vi "Send commands to manipulator.vi"(6 "read":bool, 7 "delay before read (ms)":u32, 9 "Commands (microns)":T5 {"Zcommand (nm)" min=0.0 max=25000000.0 step=62.5 format="%.1f"; "Ycommand (nm)" format="%.1f"; "Xcommand (nm)" format="%.1f"}, 10 "Manipulator":i32(ring) items=["1", "2", "3", "4"], 11 "Command":u16(ring)=1 items=["Change manipulator", "Get current position", "Go to position", "Home", "Work", "Center", "Interrupt move"]) -> (0 "Coordinates (not rounded)":T1 {"Zcoordinate (not rounded)" format="%.4f"; "Ycoordinate (not rounded)" format="%.4f"; "Xcoordinate (not rounded)" format="%.4f"}, 1 "Coordinates (microns)":T2={"Xcoordinate (microns)"=8589, "Ycoordinate (microns)"=6028, "Zcoordinate (microns)"=4319}, 2 "Coordinates (nm)":T3={"Xcoordinate (nm)"=8589.0, "Ycoordinate (nm)"=6028.0, "Zcoordinate (nm)"=4319.0} {"Xcoordinate (nm)" format="%.1f"; "Ycoordinate (nm)" format="%.1f"; "Zcoordinate (nm)" format="%.1f"}, 3 "Commands (microns)":T4 {"Zcommand (microns)" format="%.4f"; "Ycommand (microns)" format="%.4f"; "Xcommand (microns)" format="%.4f"}, 5 "Error":bool)   [LabVIEW 2010]
doc: "The Basic Serial Read and Write example performs a Serial Port Read, a Serial Port Write, or a combination of these actions. The user selects the actions (read or write) on the front panel. If both are selected, the VI will write the data first, read data, and then close the VISA session that is opened to the port. This VI will wait until the specified number of bytes is received at the port. Only the number of bytes specified will be read.\n\nINSTRUCTIONS:\n1) Select the serial resource and configuration parameters (baud rate, data bits, parity, stop bits, flow control).\n2) Select the operations to be performed. \n3) Connect the serial port to your device. If no device is available, perform a loopback test by doing one of the following. Short pins 2 and 3 on a RS-232 cable or short pin 4 to pin 8 and pin 5 to pin 9 on a RS-485/422 cable. \n4) Run the VI to see the data read. (The \"read string\" will match the \"string to write\" if a loopback test was performed.)\n\nNote: The parameters set for the serial port must match the parameters of the connected instrument or device. In this example, the bytes to read parameter specifies the number of bytes that the serial port reads. If there were more bytes at the port than the number specified in bytes to read, those bytes would not be read. Also, if you specify to read more bytes than the number of bytes actually read, you might receive a timeout error message.\n\nOn the block diagram, the Configure Serial Port VI sets the configuration parameters. The front panel displays the controls used to configure the basic parameters, such as baud rate, data bits, and parity. Constants configure the other parameters the user probably does not need set. After the VISA Configure Serial Port VI opens the VISA session and configures the port, the VI passes the VISA resource name to other VIs that perform operations on that VISA resource. The VISA Write function sends a command to the serial device and the VISA Read function returns data based on the command. The VISA Close function then closes the reference to the serial device. It is important to close the reference; otherwise communication through with that port through protocols other than VISA might not be possible."
uses:
  <vilib>/Instr/_visa.llb/VISA Configure Serial Port (Instr).vi
panel:
  in  "flow control":u16(ring) items=["None"=0, "XON/XOFF"=1, "RTS/CTS"=2, "DTR/DSR"=4]
  in  "stop bits":u16(ring)=10 items=["1.0"=10, "1.5"=15, "2.0"=20]
  out "string to write":string="C"
  out "bytes read":u32=13
  out "read string":string
  in  "parity":u16(ring) items=["None", "Odd", "Even", "Mark", "Space"]
  in  "data bits":u16=8 min=5 max=8 step=1
  in  "baud rate":u32=128000
  in  "VISA resource name":refnum<visa-resource-name>="COM3"
  # "hex display"
  # "NOTES\n-Smallest step = 1 microstep = .0625 microns = 62.5 nm\n-16 microsteps/micron\n\n-"
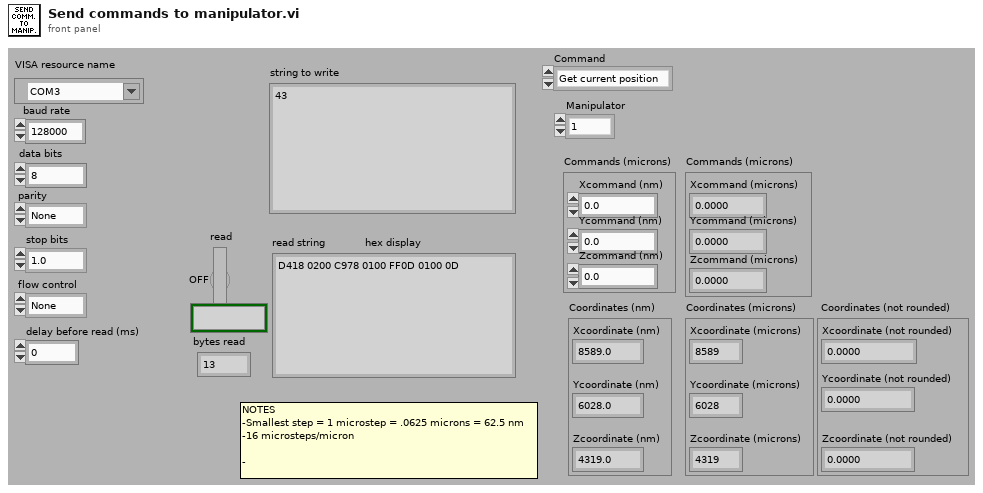
[diagram p1: front panel]
types:
  T1 = cluster{"Xcoordinate (not rounded)":dbl, "Ycoordinate (not rounded)":dbl, "Zcoordinate (not rounded)":dbl}
  T2 = cluster{"Xcoordinate (microns)":i32, "Ycoordinate (microns)":i32, "Zcoordinate (microns)":i32}
  T3 = cluster{"Xcoordinate (nm)":dbl, "Ycoordinate (nm)":dbl, "Zcoordinate (nm)":dbl}
  T4 = cluster{"Xcommand (microns)":dbl, "Ycommand (microns)":dbl, "Zcommand (microns)":dbl}
  T5 = cluster{"Xcommand (nm)":dbl, "Ycommand (nm)":dbl, "Zcommand (nm)":dbl}
  T6 = cluster{"Xcoordinate":i32, "Ycoordinate":i32, "Zcoordinate":i32}
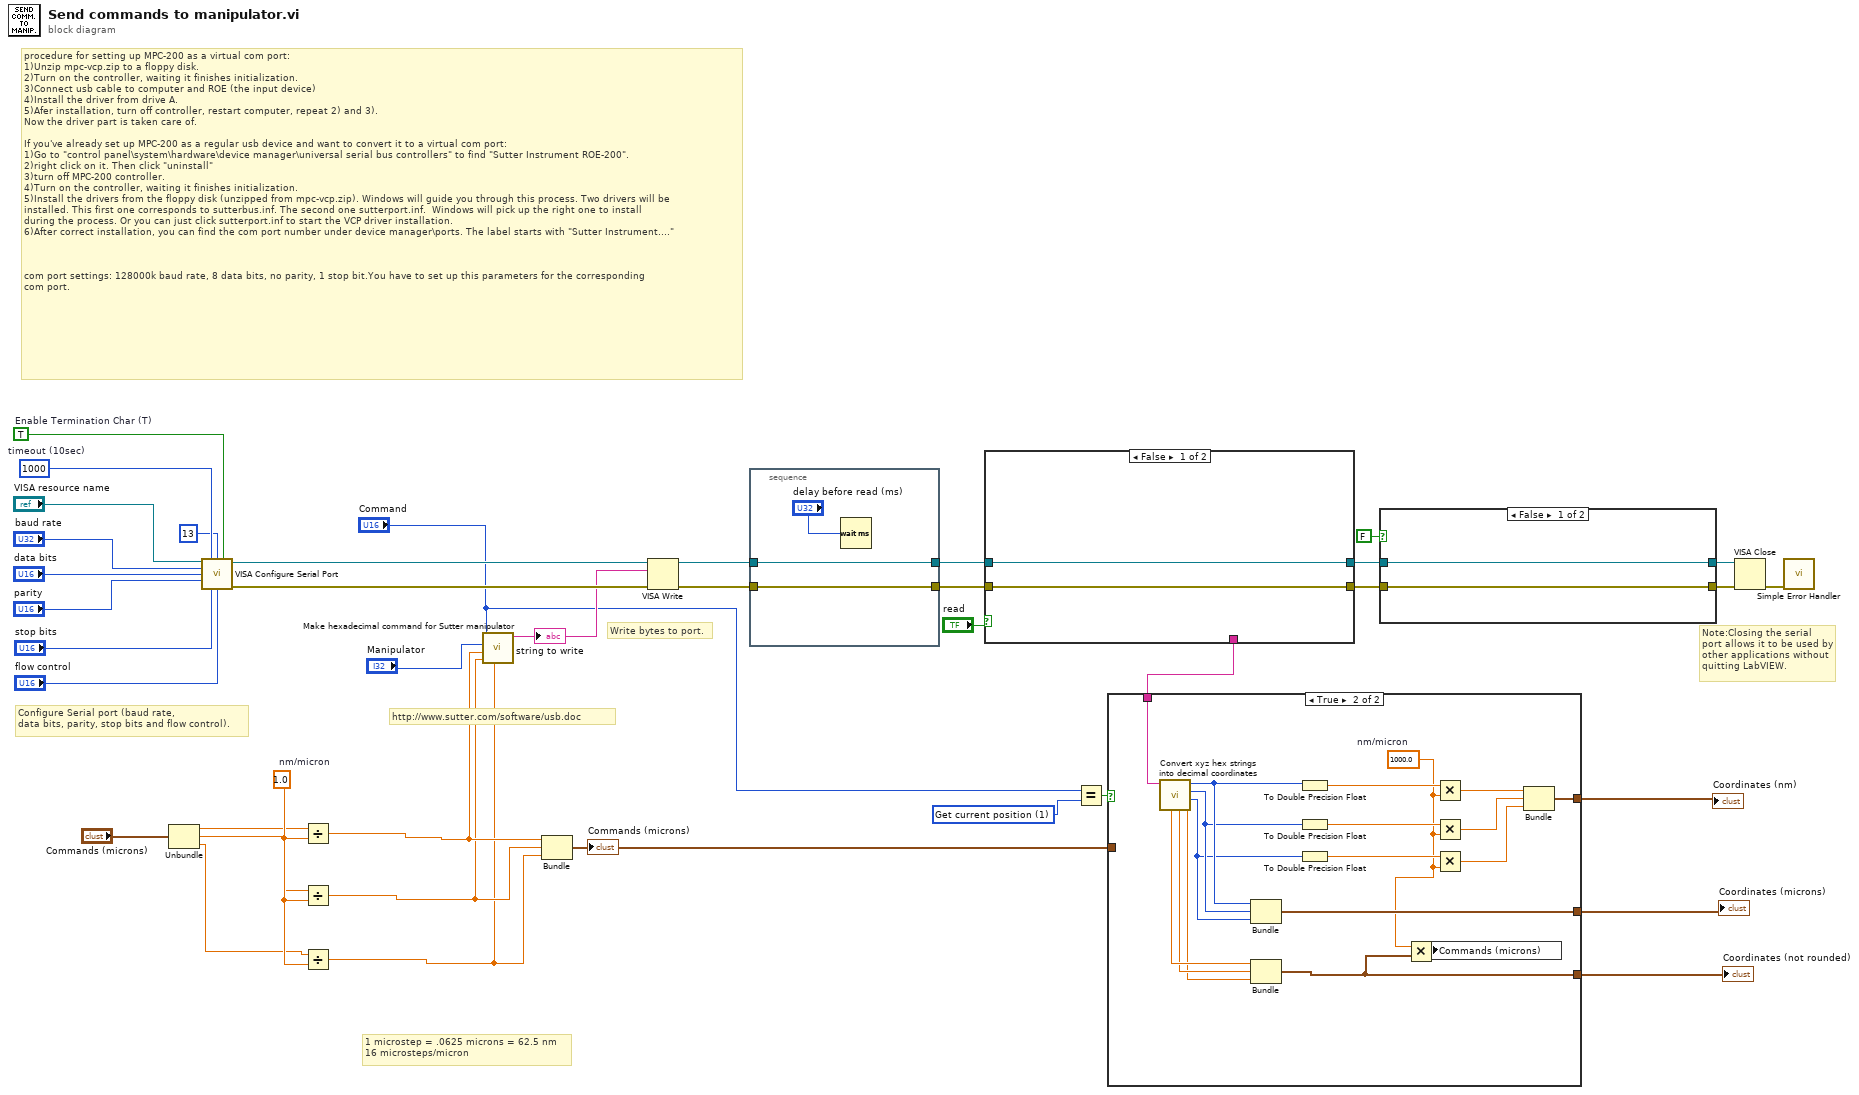
[diagram p0: block diagram]
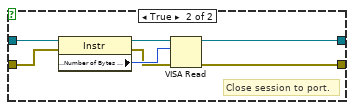
[diagram p2: hidden frame]
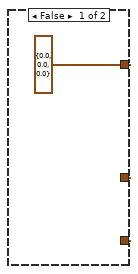
[diagram p3: hidden frame]
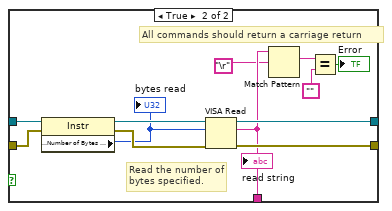
[diagram p4: hidden frame]
diagram:
  w9 = u16 1 items=["Change manipulator", "Get current position", "Go to position", "Home", "Work", "Center", "Interrupt move"] ("Command")
  w20 = 1.0  # nm/micron
  w32 = TRUE  # Enable Termination Char (T)
  w33 = u32 1000  # timeout (10sec)
  # "http://www.sutter.com/software/usb.doc"
  # "Write bytes to port."
  # "1 microstep = .0625 microns = 62.5 nm\n16 microsteps/micron"
  # "Note:Closing the serial port allows it to be used by other applications without\nquitting LabVIEW."
  # "Configure Serial port (baud rate,\ndata bits, parity, stop bits and flow control)."
  # "procedure for setting up MPC-200 as a virtual com port:\n1)Unzip mpc-vcp.zip to a floppy disk.\n2)Turn on the controller, waiting it finishes initialization.\n3)Connect usb cable to computer and ROE (the input device)\n4)Install the driver from drive A. \n5)Afer installation, turn off controller, restart computer, repeat 2) and 3).\nNow the driver part is taken care of.\n\nIf you've already set up MPC-200 as a regular usb device and want to convert it to a virtual com port:\n1)Go to \"control panel\\system\\hardware\\device manager\\universal serial bus controllers\" to find \"Sutter Instrument ROE-200\".\n2)right click on it. Then click \"uninstall\"\n3)turn off MPC-200 controller.\n4)Turn on the controller, waiting it finishes initialization.\n5)Install the drivers from the floppy disk (unzipped from mpc-vcp.zip). Windows will guide you through this process. Two drivers will be \ninstalled. This first one corresponds to sutterbus.inf. The second one sutterport.inf.  Windows will pick up the right one to install\nduring the process. Or you can just click sutterport.inf to start the VCP driver installation.\n6)After correct installation, you can find the com port number under device manager\\ports. The label starts with \"Sutter Instrument....\"\n\n\n\ncom port settings: 128000k baud rate, 8 data bits, no parity, 1 stop bit.You have to set up this parameters for the corresponding \ncom port."
  n1 = Unbundle("Commands (microns)") -> ("Xcommand (nm)"=w18:dbl, "Ycommand (nm)"=w17:dbl, "Zcommand (nm)"=w5:dbl)
  n2 = call-poly "VISA Configure Serial Port"("VISA resource name"="VISA resource name", "timeout (10sec)"=w33, "termination char\n(0xA = '\\n' = LF)"=u8 13 ("termination char\n(0xA = '\\n' = LF)"), "Enable Termination\nChar (T)"=w32, "baud rate (9600)"="baud rate", "data bits (8)"="data bits", "parity (0:none)"="parity", "stop bits (10: 1 bit)"="stop bits", "flow control (0:none)"="flow control") -> ("VISA resource name out"=w36:refnum<visa-resource-name>, "error out"=w37:errorcluster)  [unwired: 1 in, 4 out]
  n3 = Divide(x=w18, y=w20) -> (x/y=w4:dbl)
  n4 = Divide(x=w17, y=w20) -> (x/y=w3:dbl)
  n5 = Divide(x=w5, y=w20) -> (x/y=w2:dbl)
  n6 = call "Make hexadecimal command for Sutter manipulator.vi"("Zcommand (microns)"=w2, "Ycommand (microns)"=w3, "Xcommand (microns)"=w4, "Manipulator"="Manipulator", "Command"="Command") -> ("Hexadecimal command string"=w21:string)  [unwired: 6 in]
  "string to write" <- w21
  n7 = Bundle(w4, w3, w2) -> (w1:cluster{dbl, dbl, dbl})  [unwired: 1 out]
  "Commands (microns)" <- w1
  n8 = VISA Write(VISA resource name=w36, write buffer=w21, error in (no error)=w37) -> (VISA resource name out=w26:refnum<visa-resource-name>, error out=w28:errorcluster)  [unwired: 1 out]
  n9 = stacked-sequence {
    tunnel: w28 -> [w41]
    tunnel: [w41] -> w27
    tunnel: w26 -> [w42]
    tunnel: [w42] -> w25
    frame #0 {
      n10 = Wait (ms)(milliseconds to wait="delay before read (ms)") -> ()  [unwired: 1 out]
    }
  }
  n11 = case shown="False" "read" {
    tunnel: w27 -> [w45 w53]
    tunnel: [w45 w57] -> w15
    tunnel: [w44 w56] -> w16
    tunnel: w25 -> [w44 w55]
    tunnel: [_ w50] -> w23
    frame False {
    }
    frame True {
      # "All commands should return a carriage return"
      # "Read the number of bytes specified."
      n12 = property class="Instr"(reference=w55, error in=w53) -> (reference out=w54:refnum<visa-resource-name>, error out=w52:errorcluster, "Serial Settings:Number of Bytes at Serial Port"=w51:u32)
      "bytes read" <- w51
      n13 = VISA Read(VISA resource name=w54, byte count=w51, error in (no error)=w52) -> (VISA resource name out=w56:refnum<visa-resource-name>, read buffer=w50:string, error out=w57:errorcluster)  [unwired: 1 out]
      "read string" <- w50
      n14 = Match Pattern(string=w50, regular expression="\r") -> (match substring=w48:string)  [unwired: 4 out]
      n15 = Equal?(x=w48, y="") -> (x = y?=→"Error":bool)
    }
  }
  n16 = Equal?(x="Command", y=w9) -> (x = y?=w24:bool)
  n17 = case shown="True" w24 {
    tunnel: w23 -> [_ w76]
    tunnel: [w58 w63] -> w8
    tunnel: [w58 w65] -> w12
    tunnel: [w58 w62] -> w11
    tunnel: w1 -> [_ _]
    frame False {
      w58 = cluster{dbl, dbl, dbl} {0.0, 0.0, 0.0}
    }
    frame True {
      w59 = 1000.0  # nm/micron
      n18 = call "Convert xyz hex strings into decimal coordinates.vi"("read string"=w76) -> ("Zcoordinate (not rounded)"=w64:dbl, "Zcoordinate"=w73:i32, "Ycoordinate"=w74:i32, "Xcoordinate"=w75:i32, "Ycoordinate (not rounded)"=w66:dbl, "Xcoordinate (not rounded)"=w67:dbl)  [unwired: 5 in]
      n19 = Bundle("Xcoordinate"=w75, "Ycoordinate"=w74, "Zcoordinate"=w73) -> (w65:T6)  [unwired: 1 out]
      n20 = Bundle("Xcoordinate (not rounded)"=w67, "Ycoordinate (not rounded)"=w66, "Zcoordinate (not rounded)"=w64) -> (w62:T1)  [unwired: 1 out]
      n21 = To Double Precision Float(number=w75) -> (double precision float=w69:dbl)
      n22 = To Double Precision Float(number=w74) -> (double precision float=w68:dbl)
      n23 = To Double Precision Float(number=w73) -> (double precision float=w61:dbl)
      n24 = Multiply(x=w59, y=w62) -> (x*y=w60:T1)
      n25 = local write "Commands (microns)"(w60) -> ()
      n26 = Multiply(x=w69, y=w59) -> (x*y=w72:dbl)
      n27 = Multiply(x=w68, y=w59) -> (x*y=w71:dbl)
      n28 = Multiply(x=w61, y=w59) -> (x*y=w70:dbl)
      n29 = Bundle(w72, w71, w70) -> (w63:cluster{dbl, dbl, dbl})  [unwired: 1 out]
    }
  }
  "Coordinates (nm)" <- w8
  "Coordinates (microns)" <- w12
  "Coordinates (not rounded)" <- w11
  n30 = case shown="False" FALSE {
    tunnel: w16 -> [w78 w85]
    tunnel: w15 -> [w77 w84]
    tunnel: [w78 w80] -> w14
    tunnel: [w77 w79] -> w13
    frame False {
    }
    frame True {
      # "Close session to port."
      n31 = property class="Instr"(reference=w85, error in=w84) -> (reference out=w82:refnum<visa-resource-name>, error out=w81:errorcluster, "Serial Settings:Number of Bytes at Serial Port"=w83:u32)
      n32 = VISA Read(VISA resource name=w82, byte count=w83, error in (no error)=w81) -> (VISA resource name out=w80:refnum<visa-resource-name>, error out=w79:errorcluster)  [unwired: 2 out]
    }
  }
  n33 = VISA Close(VISA resource name=w14, error in (no error)=w13) -> (error out=w35:errorcluster)
  n34 = call <vilib>:"Simple Error Handler.vi"("error in (no error)"=w35) -> ()  [unwired: 1 in, 8 out]
